vi "Delete_From_Array_2D.vi"(9 "Delete from Array 2D":i8[][](array[numeric])=[[-5, -1, 3], [-4, 0, 4], [-3, 1, 5], [-2, 2, 6]], 10 "length":i32, 11 "Indexs DFA":T1={"Rows"=-1, "Columns"=-1} {"Columns" min=-1; "Rows" min=-1}) -> (1 "Deleted Portion 2D":i8[][](array[numeric]), 2 "New Array 2D":i8[][](array[numeric]))   [LabVIEW 2018]
uses:
  Controls/Rows_Columns.ctl
panel:
  out "Columns":i32
  out "Rows":i32
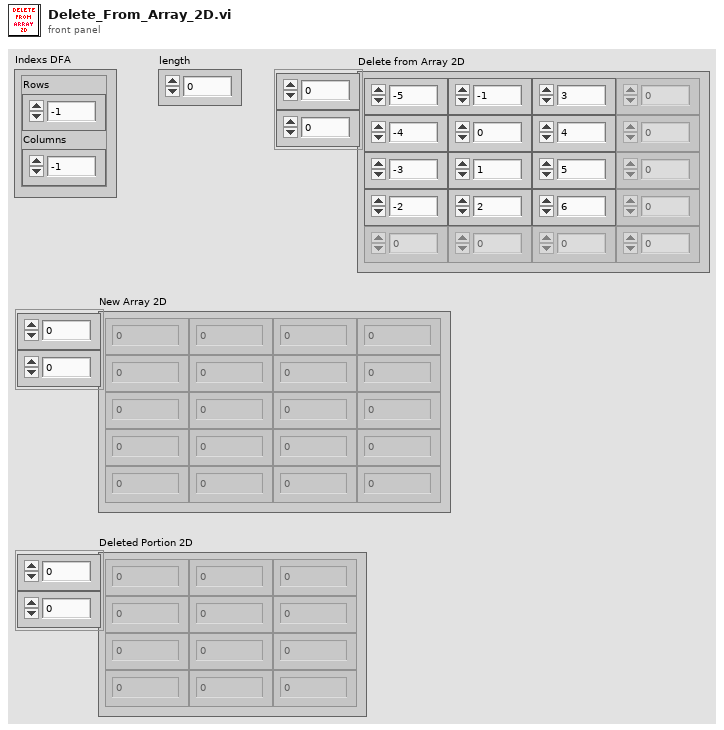
[diagram p1: front panel]
types:
  T1 = typedef "Rows_Columns.ctl" = cluster{"Rows":i32, "Columns":i32}
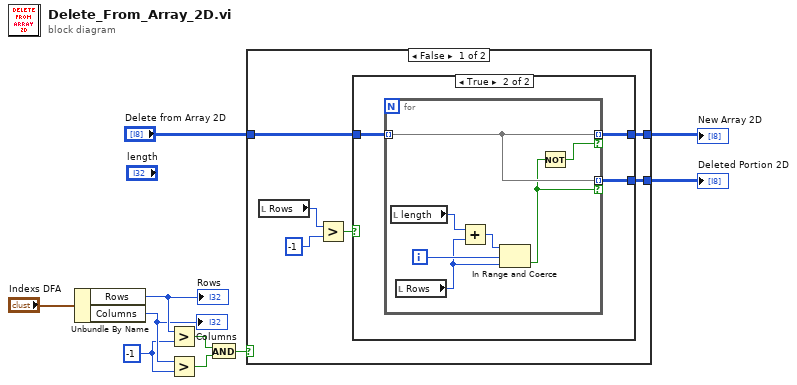
[diagram p0: block diagram]
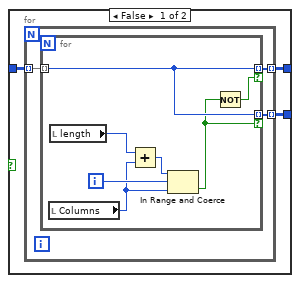
[diagram p2: hidden frame]
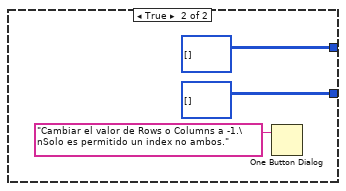
[diagram p3: hidden frame]
diagram:
  w5 = -1 ("y")
  n1 = Unbundle By Name("Indexs DFA") -> ("Rows"=w7:i32, "Columns"=w6:i32)
  "Rows" <- w7
  "Columns" <- w6
  n2 = Greater?(x=w7, y=w5) -> (0:w10:bool)
  n3 = Greater?(x=w6, y=w5) -> (0:w9:bool)
  n4 = And(x=w10, y=w9) -> (x .and. y?=w4:bool)
  n5 = case shown="False" w4 {
    tunnel: "Delete from Array 2D" -> [w13 _]
    tunnel: [w12 i8[][] [] ("Delete from Array 2D")] -> w1
    tunnel: [w11 i8[][] [] ("Delete from Array 2D")] -> w2
    frame False {
      n6 = local read "Rows"() -> (w16:i32)
      n7 = Greater?(x=w16, y=-1) -> (0:w14:bool)
      n8 = case shown="True" w14 {
        tunnel: w13 -> [w19 w32]
        tunnel: [w18 w31] -> w12
        tunnel: [w17 w30] -> w11
        frame False {
          n9 = for {
            tunnel: w19 -> [w22] mode=indexing
            tunnel: [w21] -> w18 mode=indexing
            tunnel: [w20] -> w17 mode=indexing
            n10 = for {
              tunnel: [w29] -> w21 mode=indexing if=w26
              tunnel: w22 -> [w29] mode=indexing
              tunnel: [w29] -> w20 mode=indexing if=w25
              i -> [w28]
              n11 = local read "Columns"() -> (w24:i32)
              n12 = local read "length"() -> (w27:i32)
              n13 = Add(x=w27, y=w24) -> (x+y=w23:i32)
              n14 = In Range and Coerce(upper limit=w23, x=w28, lower limit=w24) -> (In Range?=w25:bool)  [unwired: 1 out]
              n15 = Not(x=w25) -> (.not. x?=w26:bool)
            }
          }
        }
        frame True {
          n16 = for {
            tunnel: w32 -> [w35] mode=indexing
            tunnel: [w35] -> w31 mode=indexing if=w34
            tunnel: [w35] -> w30 mode=indexing if=w33
            i -> [w39]
            n17 = local read "length"() -> (w38:i32)
            n18 = local read "Rows"() -> (w37:i32)
            n19 = Add(x=w38, y=w37) -> (x+y=w36:i32)
            n20 = In Range and Coerce(upper limit=w36, x=w39, lower limit=w37) -> (In Range?=w33:bool)  [unwired: 1 out]
            n21 = Not(x=w33) -> (.not. x?=w34:bool)
          }
        }
      }
    }
    frame True {
      n22 = One Button Dialog(message="Cambiar el valor de Rows o Columns a -1.\nSolo es permitido un index no ambos.") -> ()  [unwired: 1 in, 1 out]
    }
  }
  "New Array 2D" <- w1
  "Deleted Portion 2D" <- w2
